vi "Global 1.vi"() -> ()   [LabVIEW 2017]
panel:
  out "VisionXRes":dbl
  in  "Particle Measurements (Pixels)":dbl[][](array[numeric]) format="%.2f"
  out "visionExtremeDroite":dbl
  out "visionExtremeGauche":dbl
  out "offsetcmscale":dbl
  out "offsetcmswitch":dbl
  out "Position#":dbl
  out "DistanceSwitch":dbl
  out "DistanceScaleBas":dbl
  out "DistanceScaleHaut":dbl
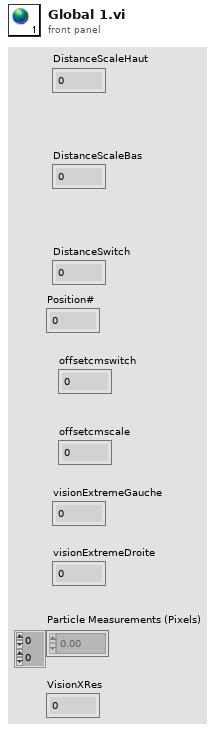
[diagram p1: front panel]
diagram:
